vi "Client.vi"(6 "timeout (ms) [500]":i32=500, 8 "error in (no error)":errorcluster, 9 "Data in":variant, 10 "Command in":variant, 11 "Instrument in":refnum<class "Instrument.lvclass">) -> (0 "error out":errorcluster, 1 "Data out":variant, 2 "Command out":string, 3 "Instrument out":refnum<class "Instrument.lvclass">)   [LabVIEW 2019, in "Instrument.lvlib" / "Instrument.lvclass"]
doc: "Remote API call via LocalClient.vi or RemoteClient.vi"
uses:
  Instrument.lvclass
  Instrument.lvclass/Instrument.ctl
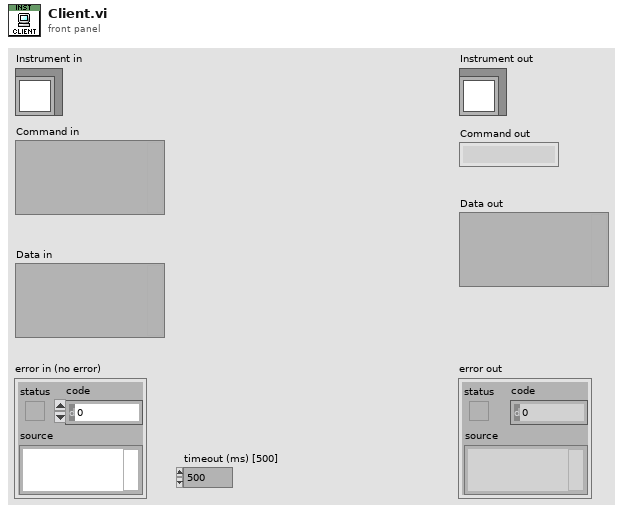
[diagram p1: front panel]
types:
  T1 = typedef "Instrument.lvlib/Instrument.lvclass/Client Type--Enum.ctl" = enum16{"Remote", "Local"}
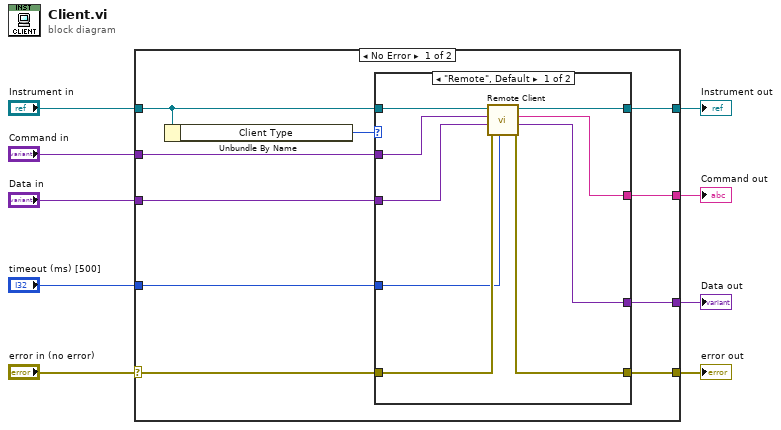
[diagram p0: block diagram]
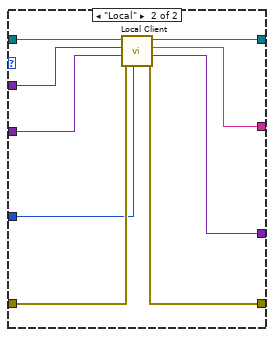
[diagram p2: hidden frame]
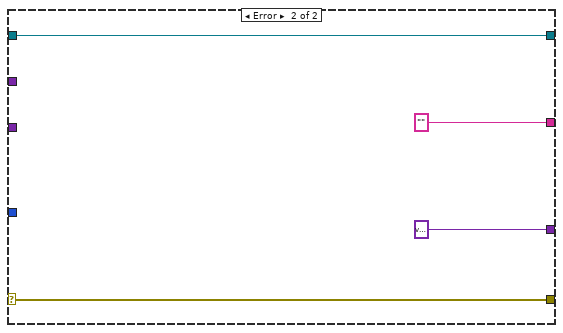
[diagram p3: hidden frame]
diagram:
  n1 = case shown="No Error" "error in (no error)" {
    selector: "error in (no error)" -> [w18 w41]
    tunnel: [w17 w41] -> w8
    tunnel: [w19 w40] -> w6
    tunnel: "Instrument in" -> [w11 w40]
    tunnel: "timeout (ms) [500]" -> [w16 _]
    tunnel: "Command in" -> [w15 _]
    tunnel: "Data in" -> [w14 _]
    tunnel: [w13 "" ("Command out")] -> w2
    tunnel: [w12 variant ("Data out")] -> w1
    frame No Error {
      n2 = Unbundle By Name(w11) -> ("Client Type"=w10:T1)
      n3 = case shown="\"Remote\", Default" w10 {
        tunnel: w11 -> [w28 w37]
        tunnel: [w27 w36] -> w19
        tunnel: w18 -> [w26 w33]
        tunnel: [w25 w32] -> w17
        tunnel: w16 -> [w24 w29]
        tunnel: w15 -> [w23 w35]
        tunnel: w14 -> [w22 w34]
        tunnel: [w21 w30] -> w13
        tunnel: [w20 w31] -> w12
        frame "Remote", Default {
          n4 = call "Remote Client.vi"("timeout (ms) [500]"=w24, "error in (no error)"=w26, "Data in"=w22, "Command in"=w23, "Instrument in"=w28) -> ("error out"=w25:errorcluster, "Data out"=w20:variant, "Command out"=w21:string, "Instrument out"=w27:refnum<class "Instrument.lvclass">)  [unwired: 3 in]
        }
        frame "Local" {
          n5 = call "Local Client.vi"("timeout (ms) [500]"=w29, "error in (no error)"=w33, "params"=w34, "Command in"=w35, "Instrument in"=w37) -> ("error out"=w32:errorcluster, "Data out"=w31:variant, "Command out"=w30:string, "Instrument out"=w36:refnum<class "Instrument.lvclass">)  [unwired: 3 in]
        }
      }
    }
    frame Error {
    }
  }
  "error out" <- w8
  "Instrument out" <- w6
  "Data out" <- w1
  "Command out" <- w2
